vi "ZMQ GEECS device publisher.vi"() -> ()   [LabVIEW 2020]
uses:
  <vilib>/addons/zeromq/socket_type.ctl
  <vilib>/addons/zeromq/zmq_context.lvclass
  <vilib>/addons/zeromq/zmq_socket.lvclass
  <vilib>/addons/zeromq/zeromq.lvlib
panel:
  in  "endpoint":string="192.168.14.2" caption="endpoint (publisher IP)"
  in  "port":i32=5555
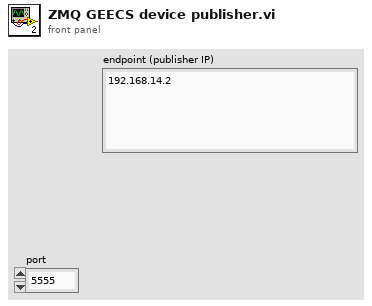
[diagram p1: front panel]
types:
  T1 = typedef "zeromq.lvlib/socket_type.ctl" = enum8{"ZMQ_PAIR", "ZMQ_PUB", "ZMQ_SUB", "ZMQ_REQ", "ZMQ_REP", "ZMQ_DEALER", "ZMQ_ROUTER", "ZMQ_PULL", "ZMQ_PUSH", "ZMQ_XPUB", "ZMQ_XSUB", "ZMQ_STREAM", "ZMQ_SERVER", "ZMQ_CLIENT", "ZMQ_RADIO", "ZMQ_DISH", "ZMQ_GATHER", "ZMQ_SCATTER", "ZMQ_DGRAM"}
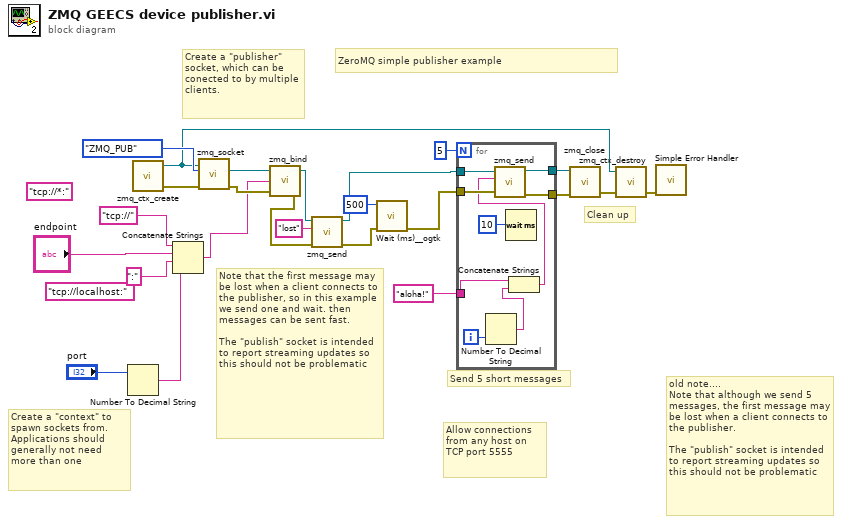
[diagram p0: block diagram]
diagram:
  (unwired) "tcp://localhost:" ("endpoint")
  (unwired) "tcp://*:" ("endpoint")
  # "Note that the first message may be lost when a client connects to the publisher, so in this example we send one and wait. then messages can be sent fast.\n\nThe \"publish\" socket is intended to report streaming updates so this should not be problematic"
  # "ZeroMQ simple publisher example"
  # "old note....\nNote that although we send 5 messages, the first message may be lost when a client connects to the publisher.\n\nThe \"publish\" socket is intended to report streaming updates so this should not be problematic"
  # "Clean up"
  # "Send 5 short messages"
  # "Allow connections from any host on TCP port 5555"
  # "Create a \"publisher\" socket, which can be conected to by multiple clients."
  # "Create a \"context\" to spawn sockets from. Applications should generally not need more than one"
  n1 = Number To Decimal String(number="port") -> (decimal integer string=w1:string)  [unwired: 1 in]
  n2 = call <vilib>:"zmq_ctx_create.vi"() -> ("error out"=w23:errorcluster, "context out"=w15:refnum<class "zmq_context.lvclass">)  [unwired: 4 in]
  n3 = Concatenate Strings("tcp://" ("endpoint"), "endpoint", ":" ("endpoint"), w1) -> (w12:string)
  n4 = call <vilib>:"zmq_socket.vi"("error in"=w23, "socket type"=socket_type."ZMQ_PUB", "context in"=w15) -> ("error out"=w22:errorcluster, "socket out"=w14:refnum<class "zmq_socket.lvclass">)  [unwired: 2 in, 1 out]
  n5 = call <vilib>:"zmq_bind.vi"("error in"=w22, "endpoint"=w12, "socket in"=w14) -> ("error out"=w8:errorcluster, "socket out"=w9:refnum<class "zmq_socket.lvclass">)  [unwired: 1 in]
  n6 = call <vilib>:"zmq_send.vi"("error in"=w8, "data"="lost", "socket in"=w9) -> ("error out"=w6:errorcluster, "socket out"=w7:refnum<class "zmq_socket.lvclass">)  [unwired: 4 in]
  n7 = call <userlib>:"Wait (ms)__ogtk.vi"("error in (no error)"=w6, "milliseconds to wait"=u32 500) -> ("error out"=w5:errorcluster)  [unwired: 8 in, 1 out]
  n8 = for {
    N: 5 -> [_]
    tunnel: w7 -> [w33]
    tunnel: w5 -> [w32]
    tunnel: [w31] -> w21
    tunnel: "aloha!" ("format string") -> [w27]
    tunnel: [w29] -> w17
    i -> [w28]
    n9 = Number To Decimal String(number=w28) -> (decimal integer string=w25:string)  [unwired: 1 in]
    n10 = Wait (ms)(milliseconds to wait=u32 10) -> ()  [unwired: 1 out]
    n11 = Concatenate Strings(w27, w25) -> (w26:string)
    n12 = call <vilib>:"zmq_send.vi"("error in"=w32, "data"=w26, "socket in"=w33) -> ("error out"=w29:errorcluster, "socket out"=w31:refnum<class "zmq_socket.lvclass">)  [unwired: 4 in]
  }
  n13 = call <vilib>:"zmq_close.vi"("error in"=w17, "socket"=w21) -> ("error out"=w18:errorcluster)  [unwired: 3 in]
  n14 = call <vilib>:"zmq_ctx_destroy.vi"("error in"=w18, "context in"=w15) -> ("error out"=w19:errorcluster)  [unwired: 3 in]
  n15 = call <vilib>:"Simple Error Handler.vi"("error in (no error)"=w19) -> ()  [unwired: 4 in, 5 out]
